vi "drum-seq-mux-pulse-test.vi"() -> ()   [LabVIEW 2019]
uses:
  <vilib>/Rock Robotics/WPI/ThirdParty/JAS_Junk/TrajLib/Enum/DrumSequence_Step_Enum.ctl
  <vilib>/Rock Robotics/WPI/ThirdParty/JAS_Junk/TrajLib/VI/Util_GetTime_U32.vi
  <vilib>/Rock Robotics/WPI/ThirdParty/JAS_Junk/TrajLib/VI/BoolCmd_Recv_Internal.vi
  <vilib>/Rock Robotics/WPI/ThirdParty/JAS_Junk/TrajLib/VI/DigSeqLogic_Edge_On.vi
  <vilib>/Rock Robotics/WPI/ThirdParty/JAS_Junk/TrajLib/VI/BoolCmd_Send_Internal.vi
  <vilib>/Rock Robotics/WPI/ThirdParty/JAS_Junk/TrajLib/VI/BoolCmd_ObtainQueue.vi
  <vilib>/Rock Robotics/WPI/ThirdParty/JAS_Junk/TrajLib/VI/Util_GetTime_U64.vi
  <vilib>/Rock Robotics/WPI/ThirdParty/JAS_Junk/TrajLib/Trajectory_Library.lvlib
panel:
  out "SEQ ACTIVE":bool
  out "All Ready":bool
  out "Error 2":bool
  out "Ready 2":bool
  out "Seq  Active 2":bool
  out "Step Number 2":T1=enum."Initialize"
  out "Output 2":bool
  out "Output 1":bool
  out "Error":bool
  out "Ready":bool
  out "Seq  Active":bool
  out "Step Number":T1=enum."Initialize"
  out "can recv":bool
  out "error out 7":errorcluster
  out "error out 6":errorcluster
  in  "seq can cmd":bool
  out "fwd recv":bool
  out "rev recv":bool
  out "error out 5":errorcluster
  out "error out 4":errorcluster
  out "error out 3":errorcluster
  out "error out 2":errorcluster
  in  "milliseconds to wait 2":u32=1000
  in  "milliseconds to wait":u32=20
  in  "seq rev cmd":bool
  in  "seq fwd cmd":bool
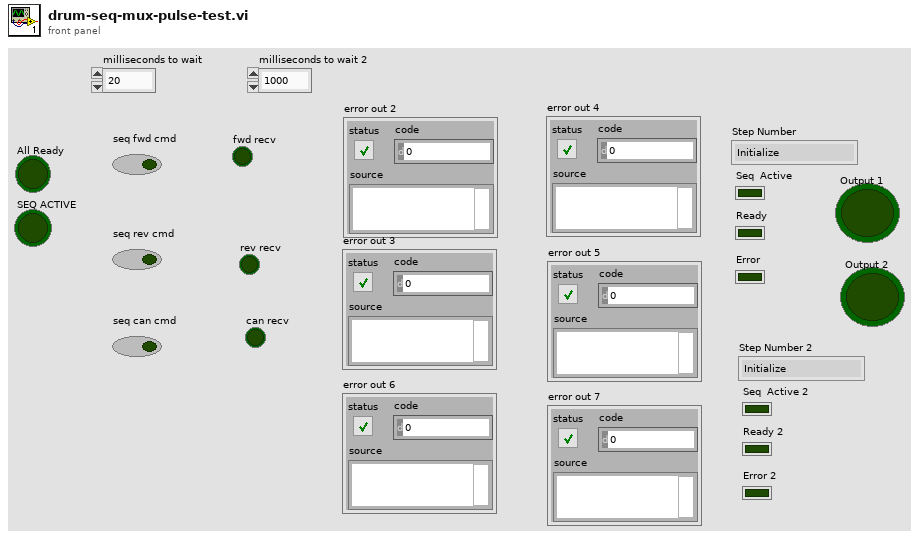
[diagram p1: front panel]
types:
  T1 = typedef "Trajectory_Library.lvlib/DrumSequence_Step_Enum.ctl" = enum16{"Do Nothing", "Step 1", "Step 2", "Step 3", "Step 4", "Step 5", "Step 6", "Step 7", "Step 8", "Step 9", "Step 10", "Step 11", "Step 12", "Step 13", "Step 14", "Step 15", "Step 16", "Step 17", "Step 18", "Step 19", "Step 20", "Step 21", "Step 22", "Step 23", "Step 24", "Step 25", "Step 26", "Step 27", "Step 28", "Step 29", "Step 30", "Step 31", "Step 32", "Cancel", "Initialize", "Error"}
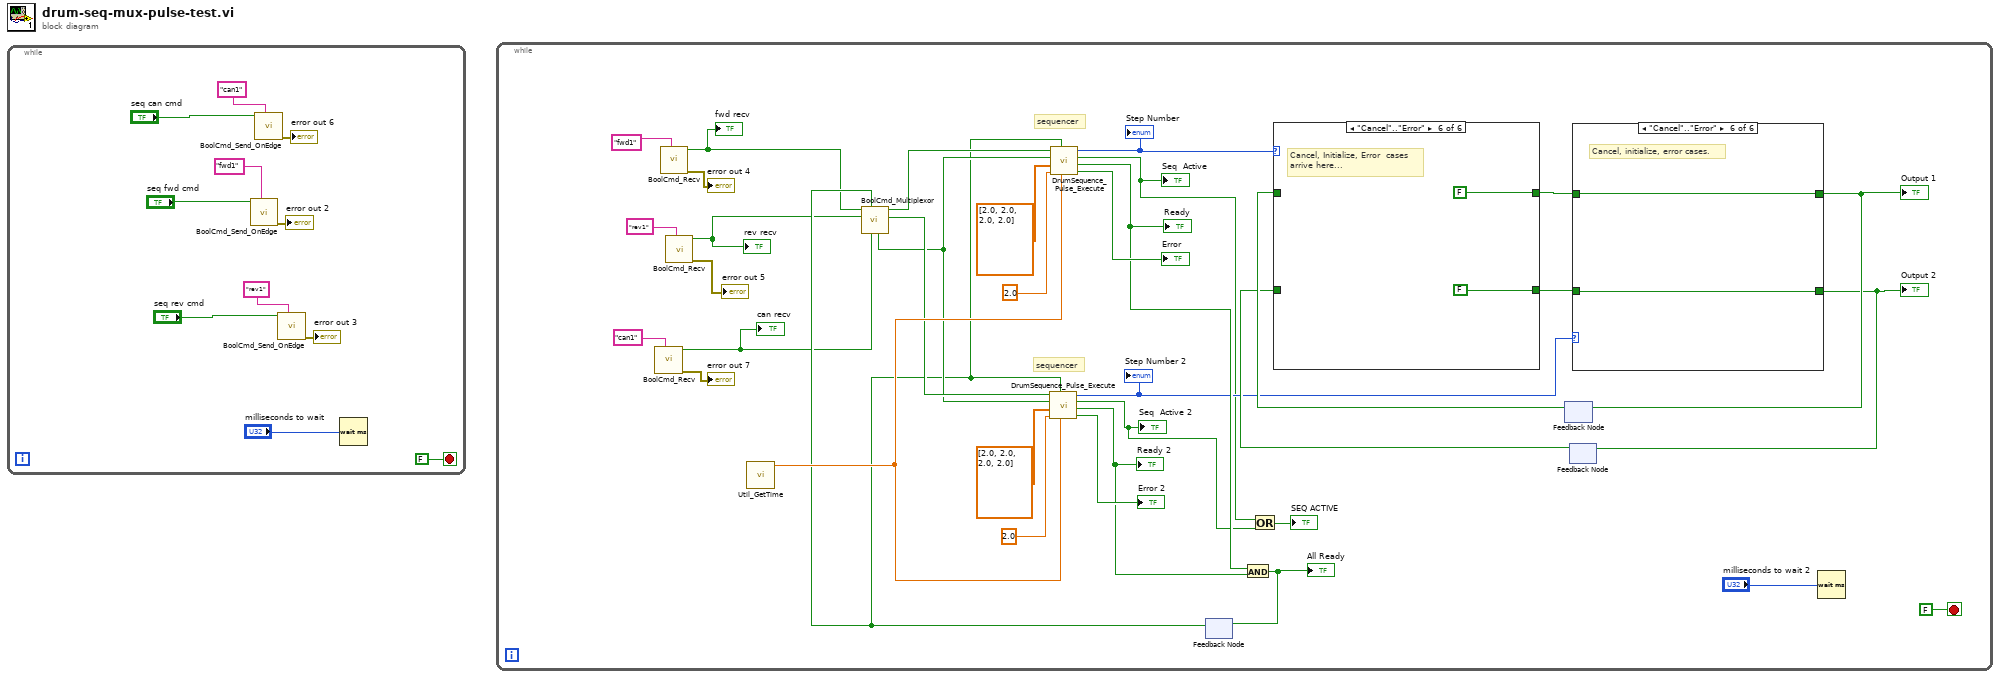
[diagram p0: block diagram]
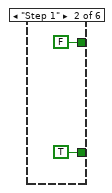
[diagram p3: hidden frame]
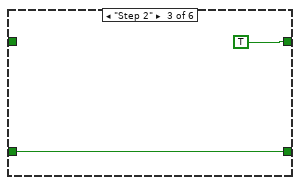
[diagram p4: hidden frame]
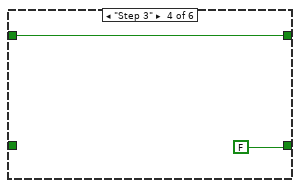
[diagram p5: hidden frame]
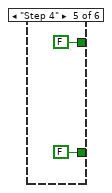
[diagram p6: hidden frame]
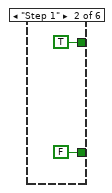
[diagram p8: hidden frame]
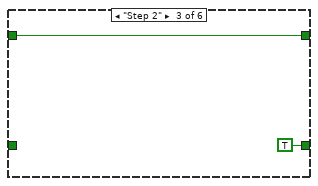
[diagram p9: hidden frame]
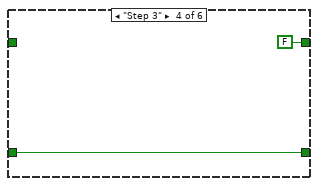
[diagram p10: hidden frame]
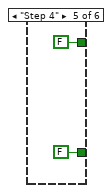
[diagram p11: hidden frame]
diagram:
  n1 = while {
    stop <- FALSE stop-if-true
    n2 = call <vilib>:"BoolCmd_Send_OnEdge.vi"("Command Name"="fwd1", "Value"="seq fwd cmd") -> ("error out"=→"error out 2":errorcluster)  [unwired: 9 in]
    n3 = call <vilib>:"BoolCmd_Send_OnEdge.vi"("Command Name"="can1", "Value"="seq can cmd") -> ("error out"=→"error out 6":errorcluster)  [unwired: 9 in]
    n4 = call <vilib>:"BoolCmd_Send_OnEdge.vi"("Command Name"="rev1", "Value"="seq rev cmd") -> ("error out"=→"error out 3":errorcluster)  [unwired: 9 in]
    n5 = Wait (ms)(milliseconds to wait="milliseconds to wait") -> ()  [unwired: 1 out]
  }
  n6 = while {
    stop <- FALSE stop-if-true
    # "sequencer"
    # "sequencer"
    n7 = call <vilib>:"BoolCmd_Recv.vi"("Command Name"="can1") -> ("error out"=→"error out 7":errorcluster, "New Request"=w12:bool)  [unwired: 9 in]
    "can recv" <- w12
    n8 = call <vilib>:"BoolCmd_Recv.vi"("Command Name"="fwd1") -> ("error out"=→"error out 4":errorcluster, "New Request"=w14:bool)  [unwired: 9 in]
    "fwd recv" <- w14
    n9 = call <vilib>:"BoolCmd_Recv.vi"("Command Name"="rev1") -> ("error out"=→"error out 5":errorcluster, "New Request"=w13:bool)  [unwired: 9 in]
    "rev recv" <- w13
    n10 = call <vilib>:"Util_GetTime.vi"() -> ("FPGA_Time_Seconds"=w19:dbl)  [unwired: 9 in, 2 out]
    n11 = feedback #1() -> (w15:bool)  [unwired: 1 in]
    n12 = call <vilib>:"BoolCmd_Multiplexor.vi"("Command Cancel"=w12, "Ready"=w15, "Command 2"=w13, "Command 1"=w14) -> ("Do Command 2"=w17:bool, "Do Command 1"=w18:bool, "Do Cancel"=w16:bool)  [unwired: 3 in, 2 out]
    n13 = call <vilib>:"DrumSequence_Pulse_Execute.vi"("Pass_Through_Time"=w19, "External Ready"=w15, "Cancel Time Sec"=2.0, "Step Times Sec"=dbl[] [2.0, 2.0, 2.0, 2.0], "Cancel"=w16, "Initiate"=w17) -> ("Error"=→"Error 2":bool, "Ready"=w25:bool, "Seq  Active"=w21:bool, "Step Number State"=w23:T1)  [unwired: 1 in, 1 out]
    "Step Number 2" <- w23
    "Seq  Active 2" <- w21
    "Ready 2" <- w25
    n14 = call <vilib>:"DrumSequence_Pulse_Execute.vi"("Pass_Through_Time"=w19, "External Ready"=w15, "Cancel Time Sec"=2.0, "Step Times Sec"=dbl[] [2.0, 2.0, 2.0, 2.0], "Cancel"=w16, "Initiate"=w18) -> ("Error"=→"Error":bool, "Ready"=w26:bool, "Seq  Active"=w22:bool, "Step Number State"=w37:T1)  [unwired: 1 in, 1 out]
    "Step Number" <- w37
    "Seq  Active" <- w22
    "Ready" <- w26
    n15 = And(x=w26, y=w25) -> (x .and. y?=w24:bool)
    "All Ready" <- w24
    n16 = feedback-in #1(w24) -> ()
    n17 = Or(x=w22, y=w21) -> (x .or. y?=→"SEQ ACTIVE":bool)
    n18 = feedback #2() -> (w35:bool)  [unwired: 1 in]
    n19 = feedback #3() -> (w34:bool)  [unwired: 1 in]
    n20 = case shown="\"Cancel\"..\"Error\"" w37 {
      tunnel: [w61 TRUE w64 FALSE FALSE FALSE] -> w33
      tunnel: [w60 FALSE TRUE w66 FALSE FALSE] -> w32
      tunnel: w35 -> [w61 _ w64 _ _ _]
      tunnel: w34 -> [w60 _ _ w66 _ _]
      frame "Do Nothing", Default {
      }
      frame "Step 1" {
      }
      frame "Step 2" {
      }
      frame "Step 3" {
      }
      frame "Step 4" {
      }
      frame "Cancel".."Error" {
        # "Cancel, Initialize, Error  cases\narrive here..."
      }
    }
    n21 = case shown="\"Cancel\"..\"Error\"" w23 {
      tunnel: [w49 FALSE TRUE w55 FALSE w59] -> w31
      tunnel: [w48 TRUE w52 FALSE FALSE w58] -> w30
      tunnel: w33 -> [w49 _ _ w55 _ w59]
      tunnel: w32 -> [w48 _ w52 _ _ w58]
      frame "Do Nothing", Default {
      }
      frame "Step 1" {
      }
      frame "Step 2" {
      }
      frame "Step 3" {
      }
      frame "Step 4" {
      }
      frame "Cancel".."Error" {
        # "Cancel, initialize, error cases."
      }
    }
    "Output 1" <- w31
    "Output 2" <- w30
    n22 = feedback-in #2(w31) -> ()
    n23 = feedback-in #3(w30) -> ()
    n24 = Wait (ms)(milliseconds to wait="milliseconds to wait 2") -> ()  [unwired: 1 out]
  }
